vi "7000string to array.vi"(4 "7170 Input":dbl[](array[numeric])) -> (1 "7000 Out":dbl[](array[numeric]))   [LabVIEW 2014]
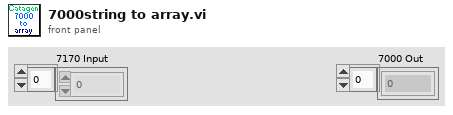
[diagram p1: front panel]
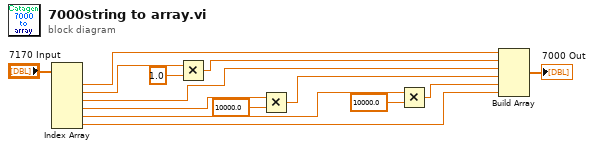
[diagram p0: block diagram]
diagram:
  n1 = Index Array(array="7170 Input") -> (element #1=w13:dbl, element #2=w7:dbl, element #3=w5:dbl, element #4=w9:dbl, element #5=w11:dbl, element #6=w2:dbl)  [unwired: 6 in]
  n2 = Multiply(x=w7, y=1.0) -> (x*y=w6:dbl)
  n3 = Multiply(x=w9, y=10000.0) -> (x*y=w4:dbl)
  n4 = Multiply(x=w11, y=10000.0) -> (x*y=w3:dbl)
  n5 = Build Array(w13, w6, w5, w4, w3, w2) -> (→"7000 Out":dbl[])
